vi "TIO Parse Packet.vi"(11 "Packet":string="\u0002\u0000\f\u0000Q\u0017\b€dev.name") -> (0 "Payload":string, 1 "Payload Length":u16, 2 "Routing Size":u8, 3 "Type":u16(ring)=2 items=["Invalid", "Log", "RPC Request", "RPC Reply", "RPC Error", "Stream Description", "User"])   [LabVIEW 2019]
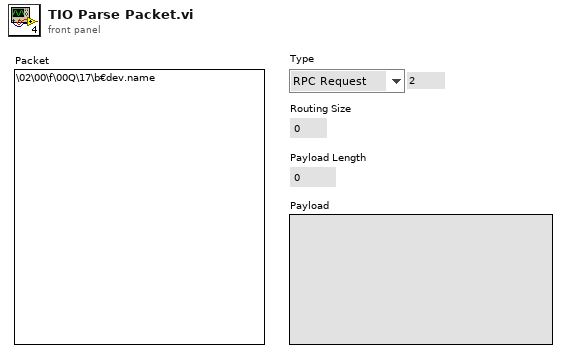
[diagram p1: front panel]
types:
  T1 = enum8{"Invalid", "Log", "RPC Request", "RPC Reply", "RPC Error", "Stream Description", "User"}
  T2 = enum16{"big-endian, network order", "native, host order", "little-endian"}
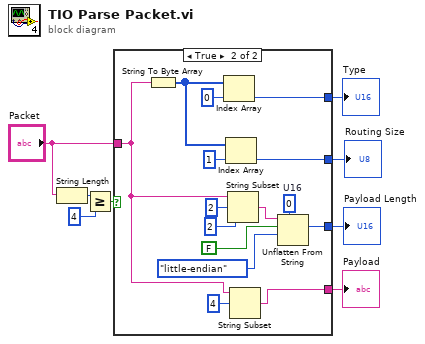
[diagram p0: block diagram]
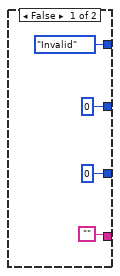
[diagram p2: hidden frame]
diagram:
  n1 = String Length(string="Packet") -> (length=w3:i32)
  n2 = Greater Or Equal?(x=w3, y=4) -> (x >= y?=w1:bool)
  n3 = case shown="True" w1 {
    tunnel: [u16 0 ("U16") w27] -> w8
    tunnel: "Packet" -> [_ w13]
    tunnel: [u8 0 w20] -> w7
    tunnel: [T1."Invalid" ("Type") w19] -> w6
    tunnel: ["" w14] -> w4
    frame False {
    }
    frame True {
      w23 = u16 0  # U16
      n4 = String To Byte Array(string=w13) -> (unsigned byte array=w22:u8[])
      n5 = Index Array(array=w22, index=0) -> (element=w19:u8)
      n6 = Index Array(array=w22, index=1) -> (element=w20:u8)
      n7 = String Subset(string=w13, offset (0)=2, length (rest)=2 ("length (rest)")) -> (substring=w26:string)
      n8 = String Subset(string=w13, offset (0)=4) -> (substring=w14:string)  [unwired: 1 in]
      n9 = Unflatten From String(type=w23, binary string=w26, data includes array or string size? (T)=FALSE, byte order (0:big-endian, network order)=T2."little-endian") -> (value=w27:u16)  [unwired: 1 in, 2 out]
    }
  }
  "Payload Length" <- w8
  "Routing Size" <- w7
  "Type" <- w6
  "Payload" <- w4
